vi "mono_send_vehicle_config.vi"(4 "error in (no error)":errorcluster, 5 "monoDrive Connection In":refnum<k5>, 7 "Vehicle Configuration Path":path=path "C:/Users/celit/Documents/GitHub/client/configurations/vehicle/demo_vehicle.json") -> (0 "error out":errorcluster, 1 "monoDrive Connection Out":refnum<k5>, 3 "vehicle command response":string)   [LabVIEW 2018, in "monoDrive.lvlib"]
uses:
  monoDrive.lvlib
  mono_config_vehicle.ctl
  mono_commands.ctl
panel:
  in  "Vehicle Configuration":T1
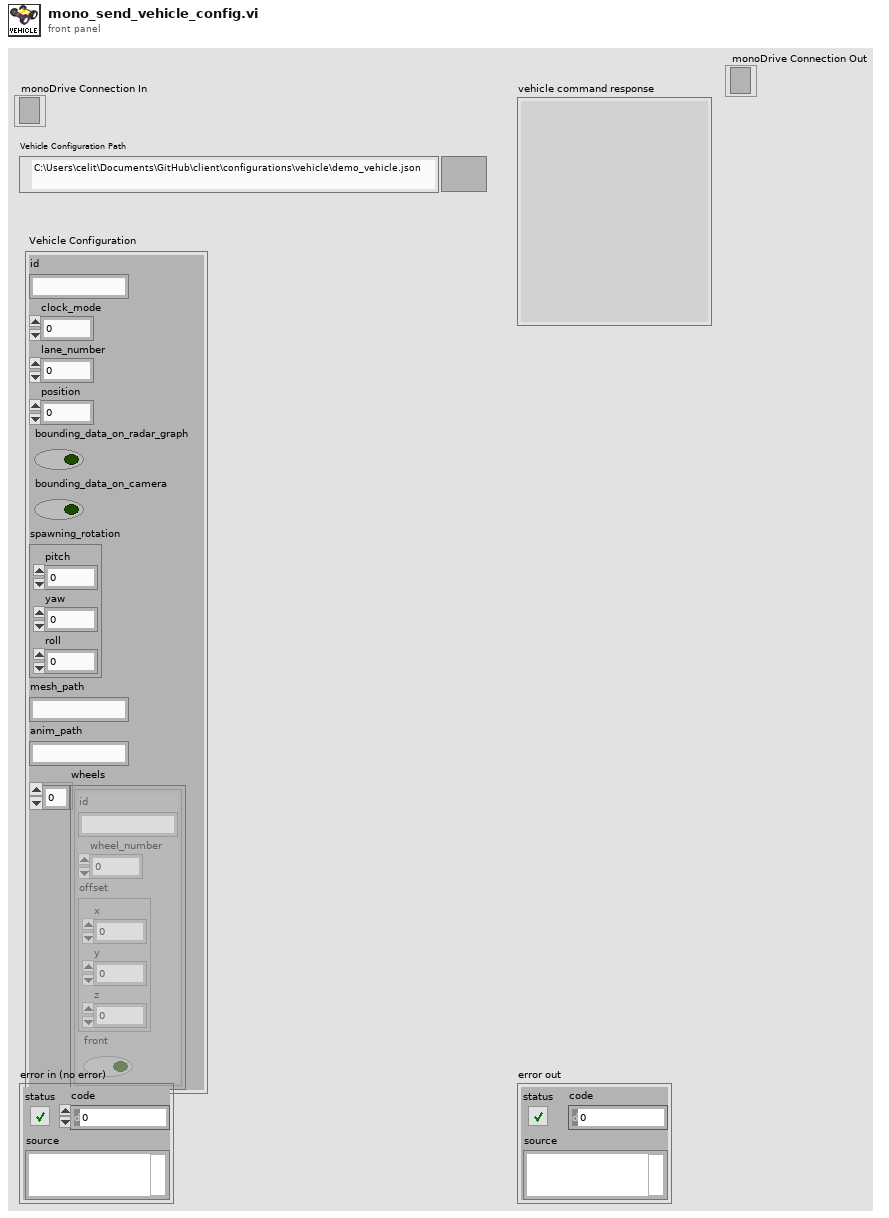
[diagram p1: front panel]
types:
  T1 = typedef "mono_config_vehicle.ctl" = cluster{"id":string, "clock_mode":i32, "lane_number":i32, "position":i32, "bounding_data_on_radar_graph":bool, "bounding_data_on_camera":bool, "spawning_rotation":cluster{"pitch":i32, "yaw":i32, "roll":i32}, "mesh_path":string, "anim_path":string, "wheels":cluster{"id":string, "wheel_number":i32, "offset":cluster{"x":i32, "y":i32, "z":i32}, "front":bool}[]}
  T2 = cluster{"type":string, "success":bool, "message":T1}
  T3 = typedef "monoDrive.lvlib/mono_commands.ctl" = cluster{"SIMULATOR_STATUS_UUID":string, "STREAM_DATA_COMMAND_UUID":string, "SIMULATOR_CONFIG_COMMAND_UUID":string, "VEHICLE_CONFIG_COMMAND_UUID":string, "EGO_CONTROL_COMMAND_UID":string, "WAYPOINT_UPDATE_COMMAND_UID":string, "SCENARIO_COMMAND_UID":string, "MAP_COMMAND_UID":string, "SPAWN_COMMAND_UID":string, "MOVE_ACTOR_COMMAND_UID":string, "SCENARIO_INIT_COMMAND_UID":string, "ATTACH_SENSOR_COMMAND_UID":string, "DETACH_SENSOR_COMMAND_UID":string, "CONTROL_HEADER":string, "RESPONSE_HEADER":string}
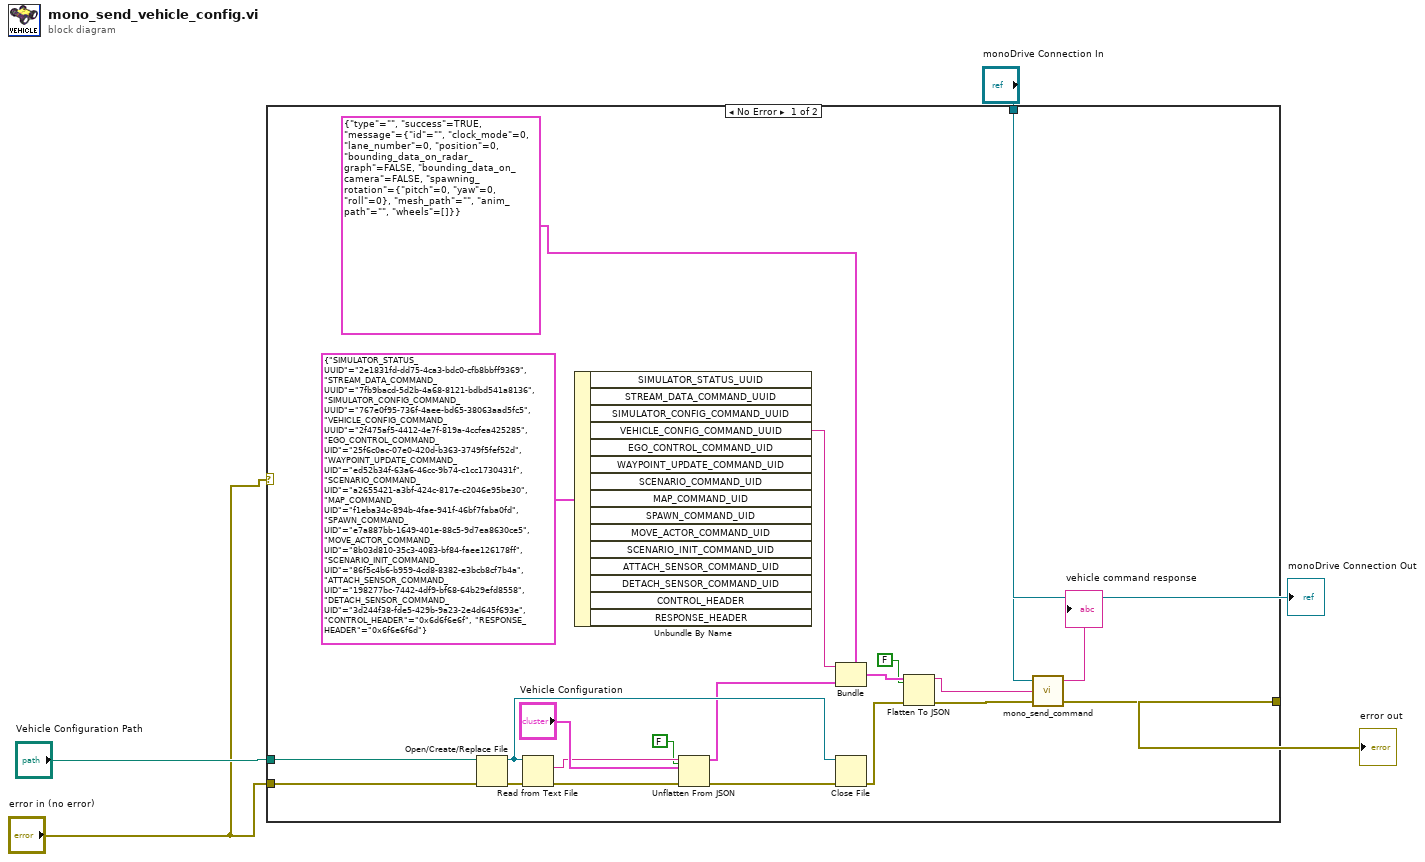
[diagram p0: block diagram]
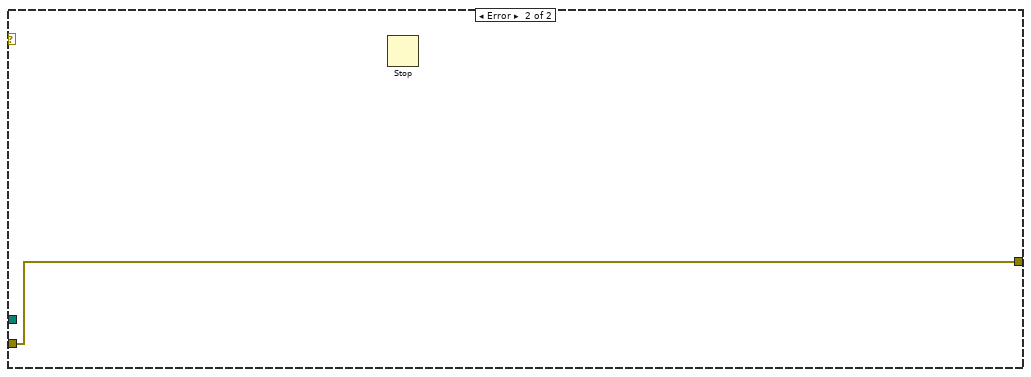
[diagram p2: hidden frame]
diagram:
  n1 = case shown="No Error" "error in (no error)" {
    tunnel: "error in (no error)" -> [w25 w26]
    tunnel: "monoDrive Connection In" -> [w23 _]
    tunnel: [w22 w26] -> w3
    tunnel: "Vehicle Configuration Path" -> [w10 _]
    frame No Error {
      n2 = Open/Create/Replace File(file path (use dialog)=w10, error in=w25) -> (refnum out=w11:refnum<file>, error out=w9:errorcluster)  [unwired: 4 in, 1 out]
      n3 = Read from Text File(file (use dialog)=w11, error in=w9) -> (text=w15:string, error out=w16:errorcluster)  [unwired: 2 in, 2 out]
      n4 = Unbundle By Name(T3 {"SIMULATOR_STATUS_UUID"="2e1831fd-dd75-4ca3-bdc0-cfb8bbff9369", "STREAM_DATA_COMMAND_UUID"="7fb9bacd-5d2b-4a68-8121-bdbd541a8136", "SIMULATOR_CONFIG_COMMAND_UUID"="767e0f95-736f-4aee-bd65-38063aad5fc5", "VEHICLE_CONFIG_COMMAND_UUID"="2f475af5-4412-4e7f-819a-4ccfea425285", "EGO_CONTROL_COMMAND_UID"="25f6c0ac-07e0-420d-b363-3749f5fef52d", "WAYPOINT_UPDATE_COMMAND_UID"="ed52b34f-63a6-46cc-9b74-c1cc1730431f", "SCENARIO_COMMAND_UID"="a2655421-a3bf-424c-817e-c2046e95be30", "MAP_COMMAND_UID"="f1eba34c-894b-4fae-941f-46bf7faba0fd", "SPAWN_COMMAND_UID"="e7a887bb-1649-401e-88c5-9d7ea8630ce5", "MOVE_ACTOR_COMMAND_UID"="8b03d810-35c3-4083-bf84-faee126178ff", "SCENARIO_INIT_COMMAND_UID"="86f5c4b6-b959-4cd8-8382-e3bcb8cf7b4a", "ATTACH_SENSOR_COMMAND_UID"="198277bc-7442-4df9-bf68-64b29efd8558", "DETACH_SENSOR_COMMAND_UID"="3d244f38-fde5-429b-9a23-2e4d645f693e", "CONTROL_HEADER"="0x6d6f6e6f", "RESPONSE_HEADER"="0x6f6e6f6d"} ("Cluster")) -> ("VEHICLE_CONFIG_COMMAND_UUID"=w14:string)  [unwired: 14 out]
      n5 = Unflatten From JSON(enable LabVIEW extensions? (T)=FALSE, JSON string=w15, type and defaults="Vehicle Configuration", error in (no error)=w16) -> (value=w5:T1, error out=w18:errorcluster)  [unwired: 3 in]
      n6 = Bundle(cluster=T2 {"type"="", "success"=TRUE, "message"={"id"="", "clock_mode"=0, "lane_number"=0, "position"=0, "bounding_data_on_radar_graph"=FALSE, "bounding_data_on_camera"=FALSE, "spawning_rotation"={"pitch"=0, "yaw"=0, "roll"=0}, "mesh_path"="", "anim_path"="", "wheels"=[]}}, "type"=w14, "message"=w5) -> (w17:T2)  [unwired: 1 in]
      n7 = Close File(refnum=w11, error in=w18) -> (error out=w24:errorcluster)  [unwired: 1 out]
      n8 = Flatten To JSON(enable LabVIEW extensions? (T)=FALSE, anything=w17, error in (no error)=w24) -> (JSON string=w20:string, 11:w21:errorcluster)
      n9 = call "mono_send_command.vi"("error in (no error)"=w21, "JSON Command"=w20, "TCP Network Connection in"=w23) -> ("error out"=w22:errorcluster, "response"=→"vehicle command response":string)  [unwired: 1 in]
    }
    frame Error {
      n10 = Stop() -> ()  [unwired: 1 in]
    }
  }
  "error out" <- w3
  "monoDrive Connection Out" <- "monoDrive Connection In"
